vi "Timestamp to ISO8601 Time.vi"(9 "UTC? (F)":bool, 11 "Timestamp (now)":timestamp) -> (3 "ISO8601 Time":string)   [LabVIEW 2024]
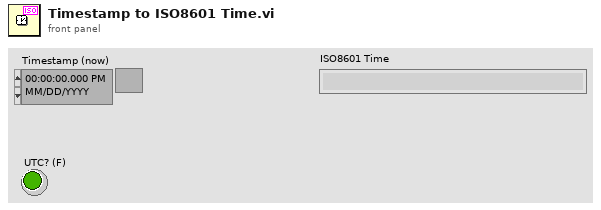
[diagram p1: front panel]
types:
  T1 = typedef "LVDateTimeRec.ctl" = cluster{"fractional second":dbl, "second":i32, "minute":i32, "hour":i32, "day of month":i32, "month":i32, "year":i32, "day of week":i32, "day of year":i32, "DST":i32}
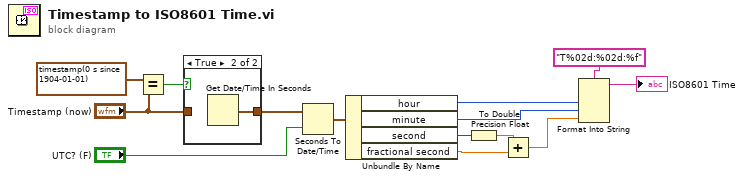
[diagram p0: block diagram]
diagram:
  n1 = Equal?(x=timestamp(0 s since 1904-01-01), y="Timestamp (now)") -> (x = y?=w9:bool)
  n2 = case shown="True" w9 {
    tunnel: [w15 w16] -> w7
    tunnel: "Timestamp (now)" -> [w15 _]
    frame False {
    }
    frame True {
      n3 = Get Date/Time In Seconds() -> (seconds since 1Jan1904=w16:timestamp)
    }
  }
  n4 = Seconds To Date/Time(time stamp (now)=w7, to UTC (F)="UTC? (F)") -> (date time rec=w11:T1)
  n5 = Unbundle By Name(w11) -> ("hour"=w6:i32, "minute"=w5:i32, "second"=w4:i32, "fractional second"=w3:dbl)
  n6 = To Double Precision Float(number=w4) -> (double precision float=w2:dbl)
  n7 = Add(x=w2, y=w3) -> (x+y=w1:dbl)
  n8 = Format Into String(format string="T%02d:%02d:%f", w6, w5, w1) -> (resulting string=→"ISO8601 Time":string)  [unwired: 2 in, 1 out]
